vi "ResetController.vi"() -> (0 "Error":bool)   [LabVIEW 2014]
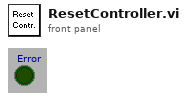
[diagram p1: front panel]
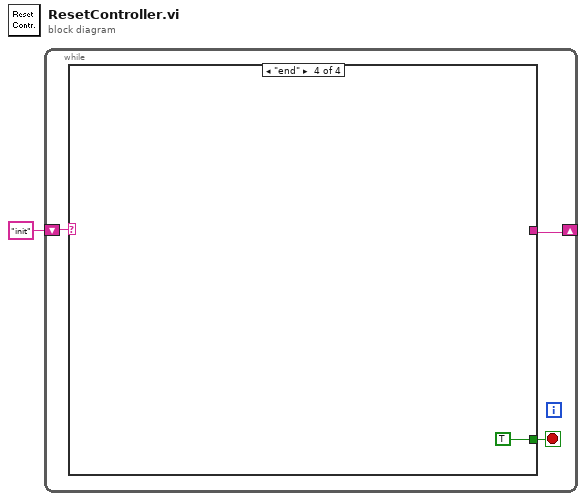
[diagram p0: block diagram]
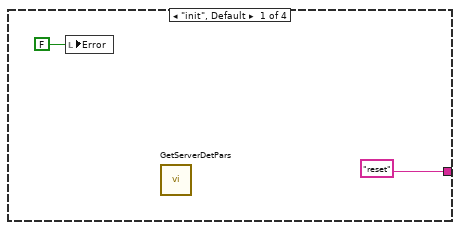
[diagram p2: hidden frame]
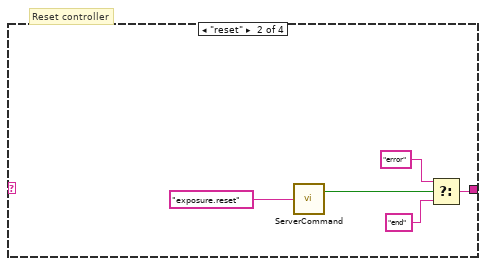
[diagram p3: hidden frame]
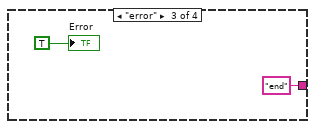
[diagram p4: hidden frame]
diagram:
  n1 = while {
    shift-right: [w2] -> _
    shift-left: "init" -> [w3]
    stop <- w4 stop-if-true
    n2 = case shown="\"end\"" w3 {
      tunnel: [_ _ _ TRUE] -> w4
      tunnel: ["reset" w9 "end" ("Error String") _] -> w2
      frame "init", Default {
        n3 = local write "Error"(FALSE ("Error")) -> ()
        n4 = call "GetServerDetPars.vi"() -> ()  [unwired: 1 in]
      }
      frame "reset" {
        # "Reset controller"
        n5 = call "ServerCommand.vi"("Command"="exposure.reset") -> ("Error"=w7:bool)  [unwired: 1 out]
        n6 = Select(t="error" ("Error String"), s=w7, f="end" ("Error String")) -> (s? t:f=w9:string)
      }
      frame "error" {
        "Error" <- TRUE ("Error")
      }
      frame "end" {
      }
    }
  }
